vi "funcionPosicion.vi"(10 "t":dbl, 11 "Cluster":T1) -> (3 "theta":dbl)   [LabVIEW 2019]
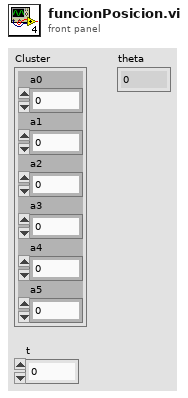
[diagram p1: front panel]
types:
  T1 = cluster{"a0":dbl, "a1":dbl, "a2":dbl, "a3":dbl, "a4":dbl, "a5":dbl}
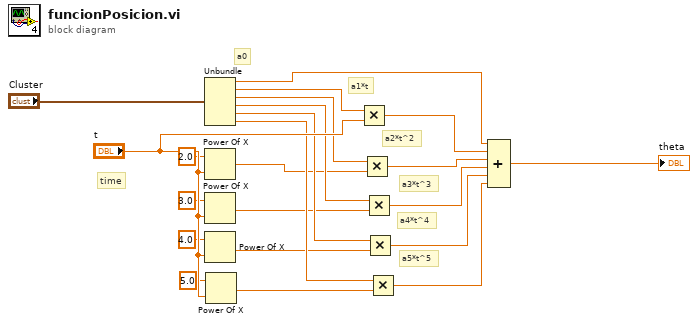
[diagram p0: block diagram]
diagram:
  # "a0"
  # "a5*t^5"
  # "a4*t^4"
  # "a3*t^3"
  # "a2*t^2"
  # "a1*t"
  # "time"
  n1 = Unbundle("Cluster") -> ("a0"=w15:dbl, "a1"=w6:dbl, "a2"=w7:dbl, "a3"=w9:dbl, "a4"=w11:dbl, "a5"=w13:dbl)
  n2 = Power Of X(1:"t", 2:2.0 ("y")) -> (0:w8:dbl)
  n3 = Power Of X(1:"t", 2:3.0 ("y")) -> (0:w10:dbl)
  n4 = Power Of X(1:"t", 2:4.0 ("y")) -> (0:w12:dbl)
  n5 = Power Of X(1:"t", 2:5.0 ("y")) -> (0:w14:dbl)
  n6 = Multiply(x=w6, y="t") -> (x*y=w16:dbl)
  n7 = Multiply(x=w7, y=w8) -> (x*y=w17:dbl)
  n8 = Multiply(x=w9, y=w10) -> (x*y=w18:dbl)
  n9 = Multiply(x=w11, y=w12) -> (x*y=w19:dbl)
  n10 = Multiply(x=w13, y=w14) -> (x*y=w20:dbl)
  n11 = Compound Arithmetic op=ADD(w15, w16, w17, w18, w19, w20) -> (→"theta":dbl)
